vi "Interlock-Objective Z.vi"() -> (3 "Cancelled":bool)   [LabVIEW 2013]
uses:
  Global Variables/gl_UI Ctrl Refs.vi
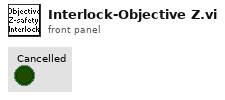
[diagram p1: front panel]
types:
  T1 = typedef "UI ctrl refs cluster.ctl" = cluster{"Top level VI path":path, "Top level VI ref":refnum<vi>, "User menu ref":refnum<k9>, "Sub Panel control":refnum<vi>, "Imaging Param Tab":refnum<vi>, "Occurrence-Start drivers":refnum<k4>, "Occurrence-Speed logging initialised":refnum<k4>, "Occurrence-XYZ stage initialised":refnum<k4>, "Exit button":refnum<vi>, "Status ind":refnum<vi>, "Return to Origin":refnum<vi>, "Speed Logging":refnum<vi>, "Time Lapse":refnum<vi>, "Live Imaging":refnum<vi>, "AOL Z Stack":refnum<vi>, "Motor Z Stack":refnum<vi>, "Funct Acq button":refnum<vi>, "Hard Shutter":refnum<vi>, "Virtual Shutter":refnum<vi>, "Laser Power":refnum<vi>, "AOL Mode":refnum<vi>, "Frame Size":refnum<vi>, "Field of View":refnum<vi>, "Dwell Time":refnum<vi>, "Zoom":refnum<vi>, "AOL Z":refnum<vi>, "Objective":refnum<vi>, "Axis":refnum<vi>, "Paths & Names":refnum<vi>, "Experiment folder path (ind.)":refnum<vi>, "Last State (Ind.)":refnum<vi>, "Laser wavelength ind (nm)":refnum<vi>, "Averages":refnum<vi>, "Angle (degrees)":refnum<vi>, "X centre":refnum<vi>, "Y centre":refnum<vi>, "Plane Mode":refnum<vi>, "# Planes":refnum<vi>, "Z Start":refnum<vi>, "Z Stop":refnum<vi>, "Z Step":refnum<vi>, "PMT 1":refnum<vi>, "PMT 2":refnum<vi>, "Stage XYZ Position":refnum<vi>, "Pockels@Z Start":refnum<vi>, "Pockels@Z Stop":refnum<vi>, "Obtain Z Start":refnum<vi>, "Obtain Z Stop":refnum<vi>, "Live stim.trig.period":refnum<vi>, "Live stim.trig.enable":refnum<vi>, "Funct. Acq. Pockels Modulation":refnum<vi>, "Enable Video Recording":refnum<vi>, "Video Record-Live Imaging":refnum<vi>, "Video Record-Funct acq":refnum<vi>, "AOL Z-stack Chirps Ready (ind)":refnum<vi>, "Center freq ind (nm)":refnum<vi>, "Logging queue (ind)":refnum<vi>, "Back aperture power (ind.)":refnum<vi>, "Power after objective (ind.)":refnum<vi>, "Switch user":refnum<vi>}
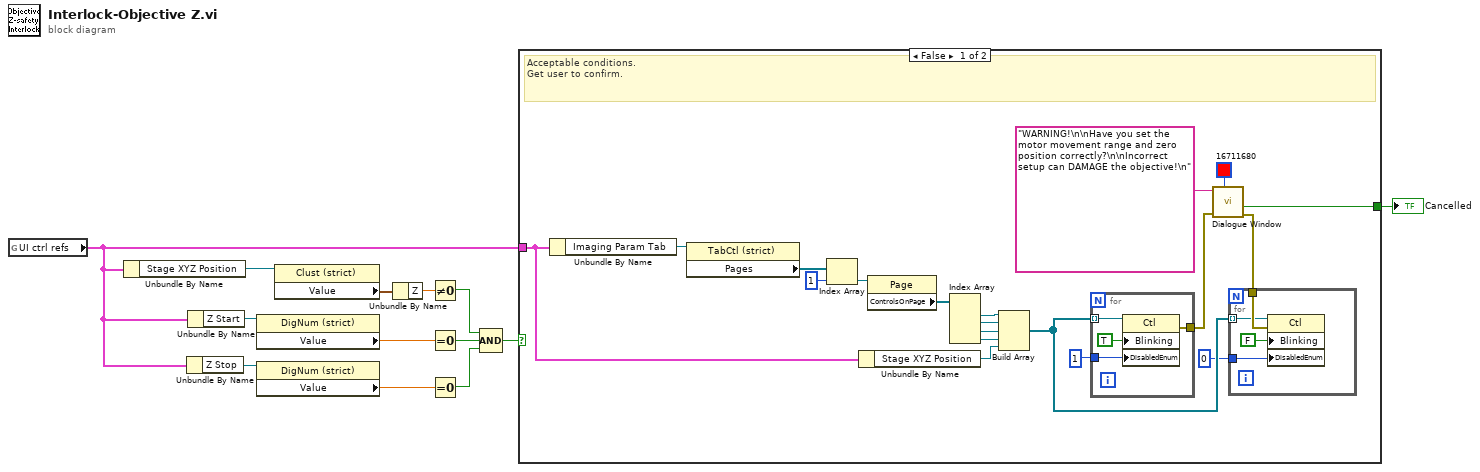
[diagram p0: block diagram]
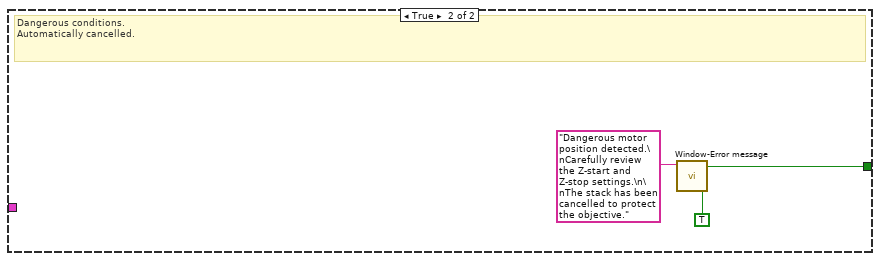
[diagram p2: hidden frame]
diagram:
  n1 = global read "gl_UI Ctrl Refs.vi" "UI ctrl refs"() -> (w1:T1)
  n2 = Unbundle By Name(w1) -> ("Stage XYZ Position"=w13:refnum<vi>)
  n3 = Unbundle By Name(w1) -> ("Z Stop"=w11:refnum<vi>)
  n4 = Unbundle By Name(w1) -> ("Z Start"=w12:refnum<vi>)
  n5 = property on="Property Node" class="DigNum (strict)"(reference=w12) -> ("Value"=w9:dbl)  [unwired: 1 in, 2 out]
  n6 = property on="Property Node" class="DigNum (strict)"(reference=w11) -> ("Value"=w8:dbl)  [unwired: 1 in, 2 out]
  n7 = property on="Property Node" class="Clust (strict)"(reference=w13) -> ("Value"=w10:cluster{"X":sgl, "Y":sgl, "Z":sgl})  [unwired: 1 in, 2 out]
  n8 = Unbundle By Name(w10) -> ("Z"=w5:sgl)
  n9 = Not Equal To 0?(x=w5) -> (x != 0?=w4:bool)
  n10 = Equal To 0?(x=w9) -> (x = 0?=w7:bool)
  n11 = Equal To 0?(x=w8) -> (x = 0?=w6:bool)
  n12 = Compound Arithmetic op=AND(w4, w7, w6) -> (w3:bool)
  n13 = case shown="False" w3 {
    tunnel: [w32 TRUE] -> w2
    tunnel: w1 -> [w15 _]
    frame False {
      # "Acceptable conditions.\nGet user to confirm."
      n14 = Unbundle By Name(w15) -> ("Imaging Param Tab"=w21:refnum<vi>)
      n15 = property class="TabCtl (strict)"(reference=w21) -> ("Pages"=w22:refnum<vi>[])  [unwired: 1 in, 2 out]
      n16 = Index Array(array=w22, index=1) -> (element=w24:refnum<vi>)
      n17 = Unbundle By Name(w15) -> ("Stage XYZ Position"=w14:refnum<vi>)
      n18 = property class="Page"(reference=w24) -> ("ControlsOnPage"=w25:refnum<vi>[])  [unwired: 1 in, 2 out]
      n19 = Index Array(array=w25) -> (element #1=w26:refnum<vi>, element #2=w27:refnum<vi>, element #3=w17:refnum<vi>, element #4=w16:refnum<vi>)  [unwired: 4 in]
      n20 = Build Array(w26, w27, w17, w16, w14) -> (w20:refnum<vi>[])
      n21 = for {
        tunnel: [w39] -> w28
        tunnel: w20 -> [w38] mode=indexing
        tunnel: 1 -> [w37]
        n22 = property class="Ctl"(reference=w38, "Blinking"=TRUE, "DisabledEnum"=w37) -> (error out=w39:errorcluster)  [unwired: 1 in, 1 out]
      }
      n23 = call "Dialogue Window.vi"("Colour"=u32 16711680 ("Color Box"), "error in (no error)"=w28, "Message string"="WARNING!\n\nHave you set the motor movement range and zero position correctly?\n\nIncorrect setup can DAMAGE the objective!\n" ("message")) -> ("error out"=w30:errorcluster, "Cancelled (Left button pressed)"=w32:bool)  [unwired: 6 in, 1 out]
      n24 = for {
        tunnel: w30 -> [w35]
        tunnel: w20 -> [w34] mode=indexing
        tunnel: 0 -> [w33]
        n25 = property class="Ctl"(reference=w34, error in=w35, "Blinking"=FALSE, "DisabledEnum"=w33) -> ()  [unwired: 2 out]
      }
    }
    frame True {
      # "Dangerous conditions.\nAutomatically cancelled."
      n26 = call "Window-Error message.vi"("Message"="Dangerous motor position detected.\nCarefully review the Z-start and Z-stop settings.\n\nThe stack has been cancelled to protect the objective." ("Message string")) -> ()  [unwired: 10 in, 1 out]
    }
  }
  "Cancelled" <- w2
